vi "HMI.vi"() -> ()   [LabVIEW 2021]
doc: "This LabVIEW project demonstrates how to use the Modbus VIs to create a set of redundant Modbus masters. In the event the primary Modbus master fails, a secondary master assumes those duties."
uses:
  Stop Global.vi
panel:
  out "Input Register Data":u16[](array[numeric])
  out "Secondary":bool
  out "Primary":bool
  out "Input Register Data (Chart)":cluster{"Numeric":u16, "Numeric":u16}(graph)
  # "Human Machine Interface (HMI)\n\nReads data from shared variables and displays the data."
  # "Master Status"
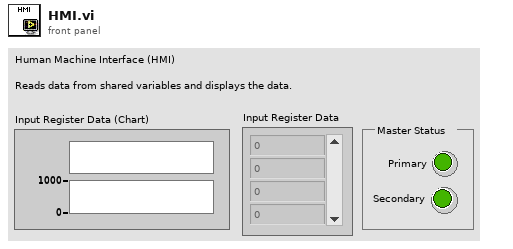
[diagram p1: front panel]
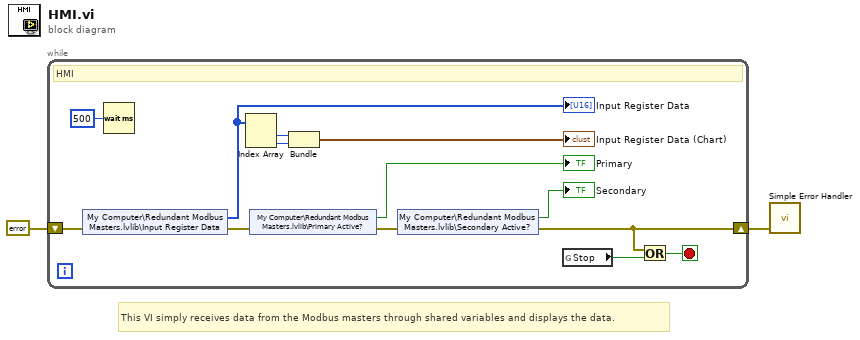
[diagram p0: block diagram]
diagram:
  # "This VI simply receives data from the Modbus masters through shared variables and displays the data."
  n1 = while {
    shift-right: [w6] -> w1
    shift-left: errorcluster {"status"=FALSE, "code"=0, "source"=""} ("error constant") -> [w7]
    stop <- w5 stop-if-true
    # "HMI"
    n2 = shared-variable "My Computer\\Redundant Modbus Masters.lvlib\\Input Register Data"(error in=w7) -> (w4:u16[], error out=w11:errorcluster)
    "Input Register Data" <- w4
    n3 = Wait (ms)(milliseconds to wait=u32 500 ("millisecond multiple")) -> ()  [unwired: 1 out]
    n4 = Index Array(array=w4) -> (element #1=w13:u16, element #2=w14:u16)  [unwired: 2 in]
    n5 = shared-variable "My Computer\\Redundant Modbus Masters.lvlib\\Primary Active?"(error in=w11) -> (→"Primary":bool, error out=w10:errorcluster)
    n6 = Bundle("Numeric"=w13, "Numeric"=w14) -> (→"Input Register Data (Chart)":cluster{"Numeric":u16, "Numeric":u16})  [unwired: 1 in]
    n7 = shared-variable "My Computer\\Redundant Modbus Masters.lvlib\\Secondary Active?"(error in=w10) -> (→"Secondary":bool, error out=w6:errorcluster)
    n8 = global read "Stop Global.vi" "Stop"() -> (w3:bool)
    n9 = Or(x=w6, y=w3) -> (x .or. y?=w5:bool)
  }
  n10 = call <vilib>:"Simple Error Handler.vi"("error in (no error)"=w1) -> ()  [unwired: 4 in, 5 out]
